vi "quiz1_programación.vi"() -> ()   [LabVIEW 2019]
panel:
  out "sum":dbl
  out "?":bool
  out "String":string
  in  "Longitud":dbl[](array[numeric])=[4.0, 1.0, 11.0, 11.0, 4.0]
  in  "Latitud":dbl[](array[numeric])=[1.0, 6.0, 14.0, 4.0, 1.0]
  in  "Py":dbl=9.0
  in  "Px":dbl=7.0
  out "Polígono":cluster{"X":dbl[], "Y":dbl[]}[](graph)
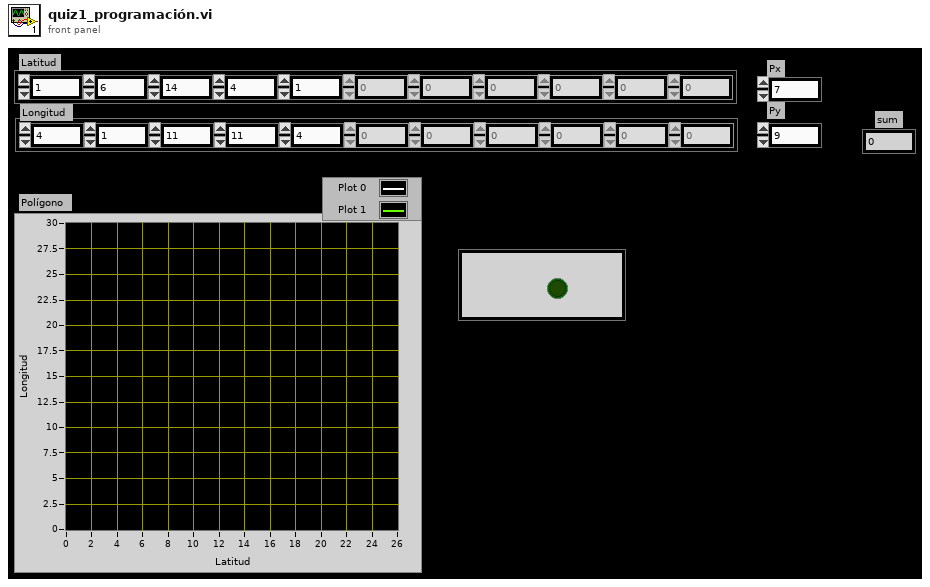
[diagram p1: front panel]
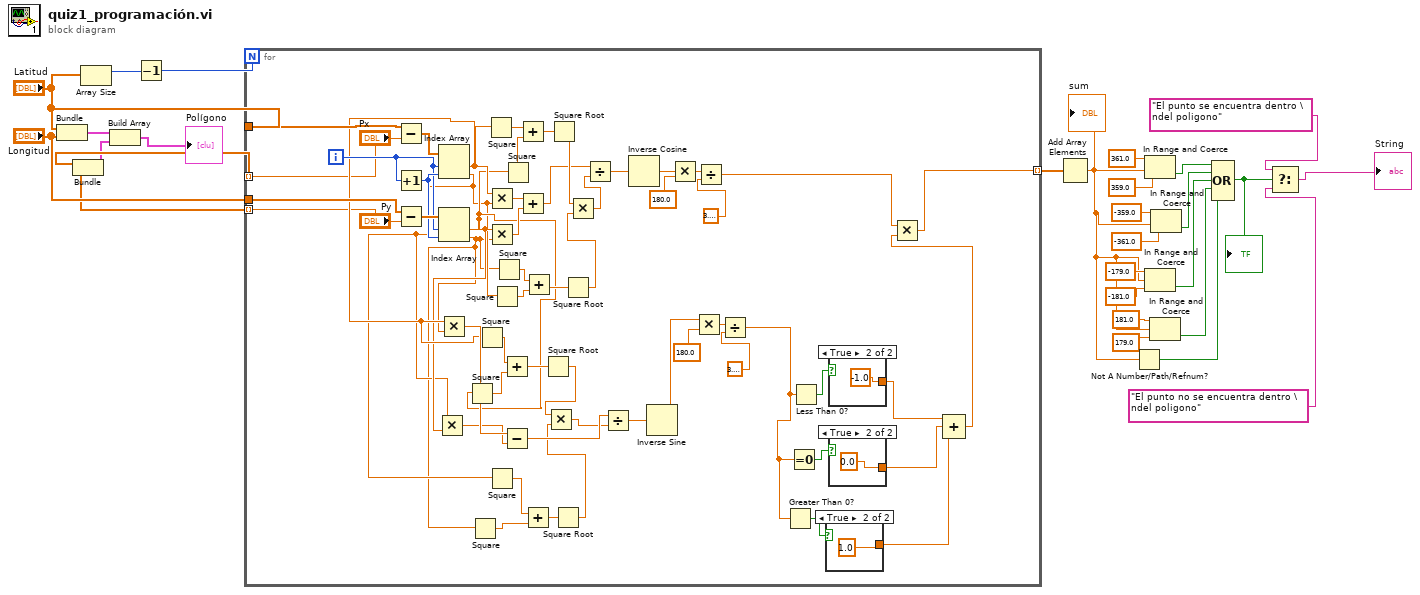
[diagram p0: block diagram]
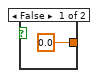
[diagram p2: hidden frame]
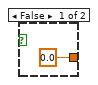
[diagram p3: hidden frame]
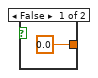
[diagram p4: hidden frame]
diagram:
  n1 = Bundle("Latitud"="Latitud", "Longitud"="Longitud") -> (w16:cluster{"Latitud":dbl[], "Longitud":dbl[]})  [unwired: 1 in]
  n2 = Array Size(array="Latitud") -> (size(s)=w26:i32)
  n3 = Decrement(x=w26) -> (x-1=w25:i32)
  n4 = for {
    N: w25 -> [_]
    tunnel: "Latitud" -> [w45]
    tunnel: "Longitud" -> [w44]
    tunnel: [w41] -> w13 mode=indexing
    tunnel: ["Px"] -> w19 mode=indexing
    tunnel: ["Py"] -> w18 mode=indexing
    i -> [w35]
    n5 = Subtract(x=w45, y="Px") -> (x-y=w84:dbl[])
    n6 = Increment(x=w35) -> (x+1=w82:i32)
    n7 = Subtract(x=w44, y="Py") -> (x-y=w83:dbl[])
    n8 = Index Array(array=w84, index #1=w35, index #2=w82) -> (element #1=w34:dbl, element #2=w32:dbl)
    n9 = Index Array(array=w83, index #1=w35, index #2=w82) -> (element #1=w33:dbl, element #2=w31:dbl)
    n10 = Multiply(x=w32, y=w33) -> (x*y=w49:dbl)
    n11 = Multiply(x=w34, y=w31) -> (x*y=w50:dbl)
    n12 = Square(x=w33) -> (x^2=w47:dbl)
    n13 = Square(x=w31) -> (x^2=w52:dbl)
    n14 = Square(x=w34) -> (x^2=w46:dbl)
    n15 = Square(x=w34) -> (x^2=w81:dbl)
    n16 = Multiply(x=w34, y=w32) -> (x*y=w77:dbl)
    n17 = Multiply(x=w33, y=w31) -> (x*y=w78:dbl)
    n18 = Square(x=w32) -> (x^2=w51:dbl)
    n19 = Square(x=w32) -> (x^2=w75:dbl)
    n20 = Square(x=w31) -> (x^2=w76:dbl)
    n21 = Add(x=w46, y=w47) -> (x+y=w48:dbl)
    n22 = Subtract(x=w50, y=w49) -> (x-y=w57:dbl)
    n23 = Square(x=w33) -> (x^2=w80:dbl)
    n24 = Add(x=w81, y=w80) -> (x+y=w79:dbl)
    n25 = Add(x=w77, y=w78) -> (x+y=w65:dbl)
    n26 = Add(x=w51, y=w52) -> (x+y=w53:dbl)
    n27 = Add(x=w76, y=w75) -> (x+y=w74:dbl)
    n28 = Square Root(x=w48) -> (sqrt(x)=w55:dbl)
    n29 = Square Root(x=w79) -> (sqrt(x)=w68:dbl)
    n30 = Square Root(x=w53) -> (sqrt(x)=w54:dbl)
    n31 = Multiply(x=w55, y=w54) -> (x*y=w56:dbl)
    n32 = Square Root(x=w74) -> (sqrt(x)=w67:dbl)
    n33 = Multiply(x=w68, y=w67) -> (x*y=w66:dbl)
    n34 = Divide(x=w65, y=w66) -> (x/y=w71:dbl)
    n35 = Divide(x=w57, y=w56) -> (x/y=w58:dbl)
    n36 = Inverse Cosine(1:w71) -> (0:w72:dbl)
    n37 = Inverse Sine(1:w58) -> (0:w38:dbl)
    n38 = Multiply(x=w72, y=180.0) -> (x*y=w73:dbl)
    n39 = Multiply(x=w38, y=180.0) -> (x*y=w40:dbl)
    n40 = Divide(x=w73, y=3.141592653589793) -> (x/y=w42:dbl)
    n41 = Divide(x=w40, y=3.141592653589793) -> (x/y=w36:dbl)
    n42 = Greater Than 0?(x=w36) -> (x > 0?=w61:bool)
    n43 = Equal To 0?(x=w36) -> (x = 0?=w60:bool)
    n44 = Less Than 0?(x=w36) -> (x < 0?=w59:bool)
    n45 = case shown="True" w61 {
      tunnel: [0.0 1.0] -> w64
      frame False {
      }
      frame True {
      }
    }
    n46 = case shown="True" w59 {
      tunnel: [0.0 -1.0] -> w62
      frame False {
      }
      frame True {
      }
    }
    n47 = case shown="True" w60 {
      tunnel: [0.0 0.0] -> w63
      frame False {
      }
      frame True {
      }
    }
    n48 = Compound Arithmetic op=ADD(w62, w63, w64) -> (w43:dbl)
    n49 = Multiply(x=w42, y=w43) -> (x*y=w41:dbl)
  }
  n50 = Bundle(w19, w18) -> (w15:cluster{dbl[], dbl[]})  [unwired: 1 in]
  n51 = Build Array(w16, w15) -> (→"Polígono":cluster{"Latitud":dbl[], "Longitud":dbl[]}[])
  n52 = Add Array Elements(numeric array=w13) -> (sum=w1:dbl)
  "sum" <- w1
  n53 = Not A Number/Path/Refnum?(number/path/refnum=w1) -> (NaN/Path/Refnum?=w2:bool)
  n54 = In Range and Coerce(upper limit=361.0, x=w1, lower limit=359.0) -> (In Range?=w22:bool)  [unwired: 1 out]
  n55 = In Range and Coerce(upper limit=-179.0, x=w1, lower limit=-181.0) -> (In Range?=w10:bool)  [unwired: 1 out]
  n56 = In Range and Coerce(upper limit=181.0, x=w1, lower limit=179.0) -> (In Range?=w3:bool)  [unwired: 1 out]
  n57 = In Range and Coerce(upper limit=-359.0, x=w1, lower limit=-361.0) -> (In Range?=w14:bool)  [unwired: 1 out]
  n58 = Compound Arithmetic op=OR(w22, w14, w10, w3, w2) -> (w9:bool)
  "?" <- w9
  n59 = Select(t="El punto se encuentra dentro \ndel poligono", s=w9, f="El punto no se encuentra dentro \ndel poligono") -> (s? t:f=→"String":string)
